vi "Conversor F a C.vi"(0 "Temperatura a convertir":dbl) -> (2 "Temperatura convertida a F":dbl)   [LabVIEW 2013]
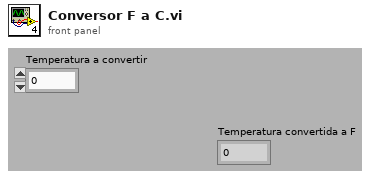
[diagram p1: front panel]
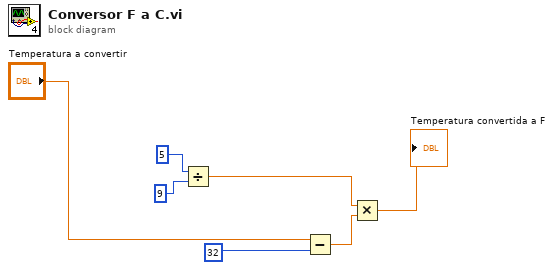
[diagram p0: block diagram]
diagram:
  n1 = Divide(x=5, y=9) -> (x/y=w3:dbl)
  n2 = Subtract(x="Temperatura a convertir", y=32) -> (x-y=w5:dbl)
  n3 = Multiply(x=w3, y=w5) -> (x*y=→"Temperatura convertida a F":dbl)
